vi "Power Supply.vi"(8 "error in (no error)":errorcluster, 11 "Power Supply in":refnum<class "Power Supply.lvclass">) -> (0 "error out":errorcluster, 3 "Power Supply out":refnum<class "Power Supply.lvclass">)   [LabVIEW 2009, in "Power Supply.lvclass"]
uses:
  Power Supply.lvclass
  Global/GPIB Numbers.vi
  Power Supply.lvclass/Power Supply.ctl
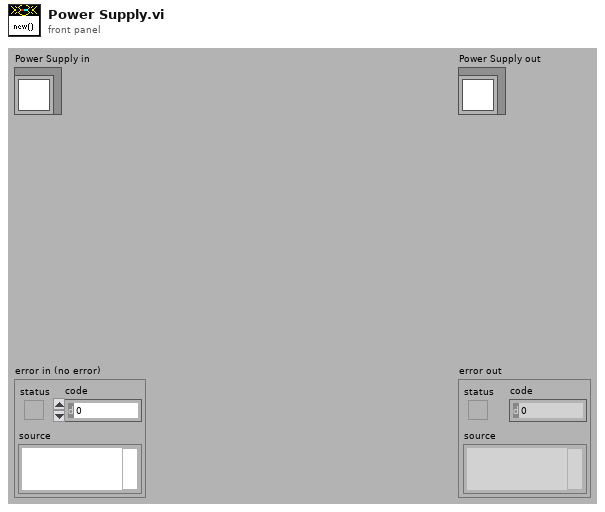
[diagram p1: front panel]
types:
  T1 = typedef "GPIB Type Def.ctl" = cluster{"Name":string, "bus":dbl, "GPIB":dbl, "GPIB as string":string, "byte":i32, "VISA Resource Name":refnum<visa-resource-name>}
  T2 = typedef "PSIO.ctl" = cluster{"Address":T3, "Version":enum16{"PS", "IPS"}}
  T3 = typedef "OxfordAddress.ctl" = cluster{"Com Port":i32, "ISOBUS Address":i32, "GPIB Address":i16, "Communication":enum16{"RS232", "ISOBUS", "GPIB", "Gateway"}}
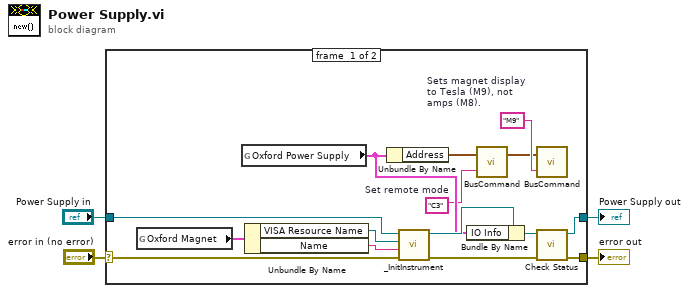
[diagram p0: block diagram]
diagram:
  n1 = case shown="No Error" "error in (no error)" {
    selector: "error in (no error)" -> [w13 w21]
    tunnel: [w10 w21] -> w3
    tunnel: [w12 w20] -> w1
    tunnel: "Power Supply in" -> [w19 w20]
    frame #0 {
      w6 = "C3"  # Set remote mode
      w8 = "M9"  # Sets magnet display to Tesla (M9), not  amps (M8).
      n2 = global read "GPIB Numbers.vi" "Oxford Magnet"() -> (w16:T1)
      n3 = global read "GPIB Numbers.vi" "Oxford Power Supply"() -> (w9:T2)
      n4 = Unbundle By Name(w16) -> ("VISA Resource Name"=w15:refnum<visa-resource-name>, "Name"=w14:string)
      n5 = Unbundle By Name(w9) -> ("Address"=w7:T3)
      n6 = call-dynamic "_InitInstrument.vi"("error in (no error)"=w13, "Name"=w14, "VISA Resource Name"=w15, "Instrument in"=w19) -> ("error out"=w11:errorcluster, "Instrument out"=w17:refnum<class "Power Supply.lvclass">)  [unwired: 6 in]
      n7 = Bundle By Name(cluster=w17, "IO Info"=w9) -> (w18:refnum<class "Power Supply.lvclass">)
      n8 = call "BusCommand.vi"("Command"=w6, "Instrument address (in)"=w7) -> ("Instrument address (out)"=w5:T3)  [unwired: 1 out]
      n9 = call "BusCommand.vi"("Command"=w8, "Instrument address (in)"=w5) -> ()  [unwired: 2 out]
      n10 = call-dynamic "Check Status.vi"("error in (no error)"=w11, "Power Supply in"=w18) -> ("error out"=w10:errorcluster, "Power Supply out"=w12:refnum<class "Power Supply.lvclass">)  [unwired: 6 in, 2 out]
    }
    frame #1 {
    }
  }
  "error out" <- w3
  "Power Supply out" <- w1
